vi "RT Error Handler - Watchdog.vi"(8 "error in (no error)":errorcluster, 10 "watchdog status":T1, 11 "Message Queue":refnum<queue>) -> (3 "dup Message Queue":refnum<queue>)   [LabVIEW 2017]
uses:
  support/Message Queue/Message Cluster.ctl
  <vilib>/RTwatchdog.llb/Watchdog status enum.ctl
  support/Message Queue/Message Queue.lvlib
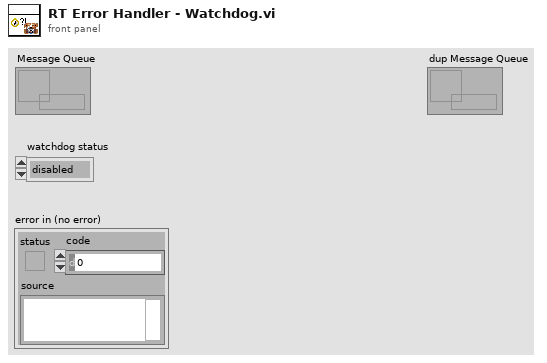
[diagram p1: front panel]
types:
  T1 = typedef "Watchdog status enum.ctl" = enum16{"disabled", "expired", "running"}
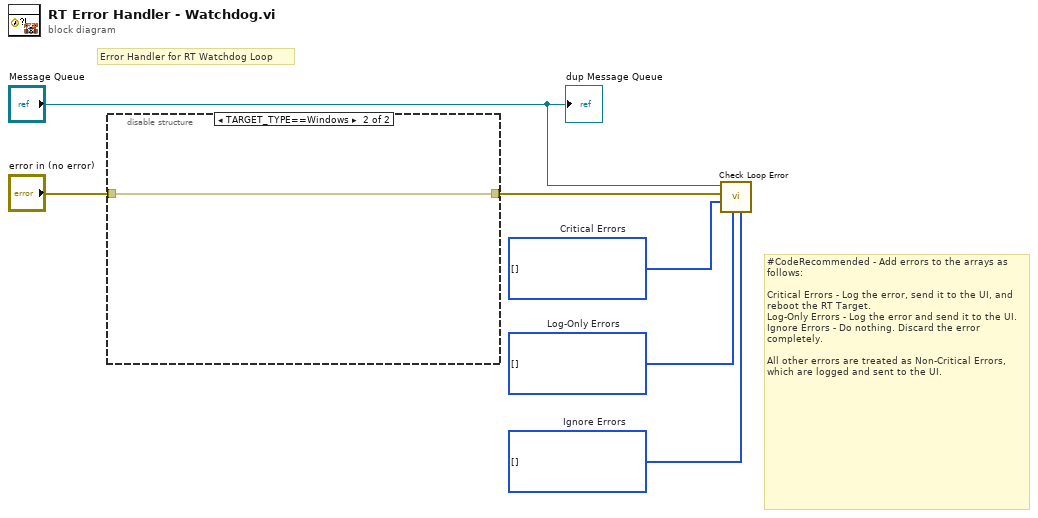
[diagram p0: block diagram]
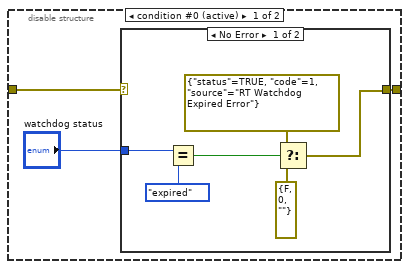
[diagram p2: hidden frame]
diagram:
  w4 = i32[] []  # Ignore Errors
  w5 = i32[] []  # Log-Only Errors
  w6 = i32[] []  # Critical Errors
  # "#CodeRecommended - Add errors to the arrays as follows:\n\nCritical Errors - Log the error, send it to the UI, and reboot the RT Target.\nLog-Only Errors - Log the error and send it to the UI.\nIgnore Errors - Do nothing. Discard the error completely.\n\nAll other errors are treated as Non-Critical Errors, which are logged and sent to the UI."
  # "Error Handler for RT Watchdog Loop"
  n1 = disable-structure shown="TARGET_TYPE==Windows" {
    disable-tunnel: "error in (no error)" -> [w9 w17]
    disable-tunnel: [w8 w17] -> w1
    frame condition #0 (active) {
      n2 = case shown="No Error" w9 {
        selector: w9 -> [_ w16]
        tunnel: [w11 w16] -> w8
        tunnel: "watchdog status" -> [w15 _]
        frame No Error {
          n3 = Equal?(x=w15, y=Watchdog_status_enum."expired") -> (x = y?=w13:bool)
          n4 = Select(t=errorcluster {"status"=TRUE, "code"=1, "source"="RT Watchdog Expired Error"} ("error constant"), s=w13, f=errorcluster {"status"=FALSE, "code"=0, "source"=""} ("error constant")) -> (s? t:f=w11:errorcluster)
        }
        frame Error {
        }
      }
    }
    frame condition #1 {
    }
  }
  n5 = call "Check Loop Error.vi"("Ignore Errors"=w4, "Log-Only Errors"=w5, "Critical Errors"=w6, "error to process"=w1, "Message Queue"="Message Queue") -> ()  [unwired: 5 in, 2 out]
  "dup Message Queue" <- "Message Queue"
